vi "Save_Info.vi"(8 "error in (no error)":errorcluster, 11 "AB_InteropAssembly in":refnum<class "AB_InteropAssembly.lvclass">) -> (0 "error out":errorcluster, 3 "AB_InteropAssembly out":refnum<class "AB_InteropAssembly.lvclass">)   [LabVIEW 2020, in "AB_InteropAssembly.lvclass"]
uses:
  <vilib>/AppBuilder/AB_Classes/InteropAssembly/AB_InteropAssembly.lvclass
  e:/builds/penguin/labview/branches/2020/dev/dist/vi.lib/AppBuilder/AB_Classes/Build/AB_Build.lvclass
  <vilib>/AppBuilder/RW_Project/AB_RW_Project_PropBag_Action.ctl
  <vilib>/AppBuilder/AB_Classes/InteropAssembly/AB_InteropAssembly.lvclass/AB_InteropAssembly.ctl
  <vilib>/AppBuilder/AB_Classes/Application/AB_Application.lvclass
  <vilib>/AppBuilder/AB_Classes/Build/AB_Build.lvclass
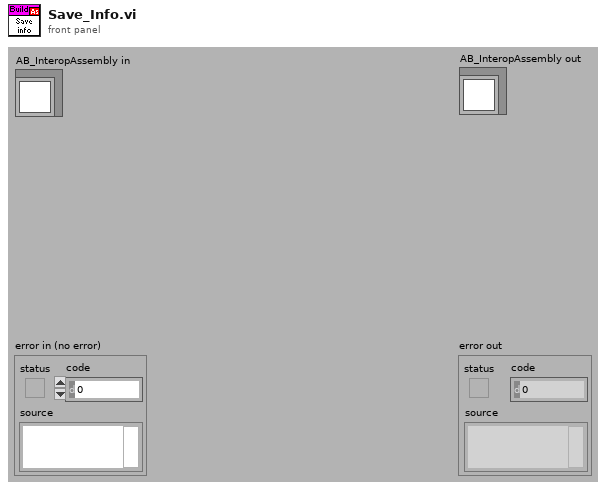
[diagram p1: front panel]
types:
  T1 = typedef "AB_RW_Project_PropBag_Action.ctl" = enum16{"read", "write", "clear", "readPrevious", "writePrevious", "clearPrevious"}
  T2 = typedef "AB_InteropAssembly.ctl" = cluster{"delayOSMsg":bool, "embeddedRTE":bool, "Namespace":string, "ClassName":string, "StrongNameKeyFilePath":path, "signAssembly":bool, "StrongNameKeyFileItemID":string, "StrongNameKeyFileGUID":string, "LabVIEW 2011 Compatibility mode":bool}
  T3 = typedef "AB_Build.ctl" = cluster{"buildSpecName":string, "buildSpecDescription":string, "destinations":refnum<class "AB_Destination.lvclass">[], "exclusionOption":T4, "defaultLanguage":string, "supportedLanguages":string[], "excludedDirectories":path[], "buildContext":refnum<vi>, "buildObject":T5, "preview":bool, "programatic":bool, "progressBarEvents":T6, "userLog_Path":path, "preActionID":string, "preAction_Path":path, "postActionID":string, "postAction_Path":path, "eng_checkForBrokenVIs?":bool, "eng_verboseLinkerErrors?":bool, "localDest_Path":path, "targetDest_Path":path, "removeVIObject":u16, "cache":refnum<class "PreviewCache.lvclass">, "use cache":bool, "previewCache_ID":string, "buildCache_ID":string, "eng_TempLocalDest_Path":path, "eng_collectDependencies?":bool, "versionInfo":cluster{"buildVersion":cluster{"major":u16, "minor":u16, "patch":u16, "build":u16}, "autoIncrement":bool}, "eng_enableVIChecksums":bool}
  T4 = typedef "AB_Exclusion_Option.ctl" = cluster{"typedefs":bool, "polymorphicVIs":bool, "unusedLibraryItems":bool, "modifyLibraryFile":bool, "edit-timeDependencies":bool, "inlineVIs":bool, "dependent PPLs":bool, "dependent DLLs":bool}
  T5 = typedef "ItemRef.ctl" = u64
  T6 = typedef "provcom_ProgressBar_Events.ctl" = cluster{"newJob":refnum<user-event>, "newItem":refnum<user-event>, "errorMsg":T7, "cancel":refnum<user-event>}
  T7 = typedef "mxLvBuildError.ctl" = refnum<user-event>
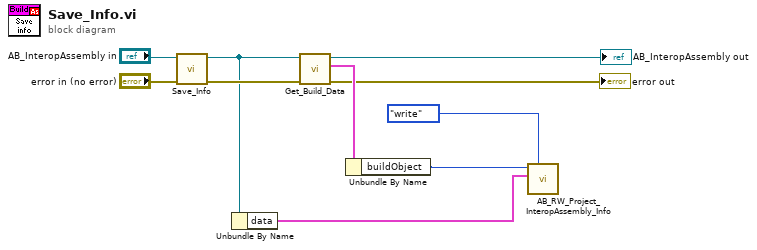
[diagram p0: block diagram]
diagram:
  n1 = call-parent "Save_Info.vi"("error in (no error)"="error in (no error)", "AB_Application in"="AB_InteropAssembly in") -> ("error out"=w8:errorcluster, "AB_Application out"=w6:refnum<class "AB_InteropAssembly.lvclass">)  [unwired: 8 out]
  n2 = Unbundle By Name(w6) -> ("data"=w2:T2)
  n3 = call <vilib>:"Get_Build_Data.vi"("error in (no error)"=w8, "Class in"=w6) -> ("error out"=→"error out":errorcluster, "data"=w9:T3, "Class out"=→"AB_InteropAssembly out":refnum<class "AB_InteropAssembly.lvclass">)  [unwired: 7 out]
  n4 = Unbundle By Name(w9) -> ("buildObject"=w1:T5)
  n5 = call <vilib>:"AB_RW_Project_InteropAssembly_Info.vi"("action"=AB_RW_Project_PropBag_Action."write", "InteropAssebly info in"=w2, "Object In"=w1) -> ()  [unwired: 1 in, 8 out]
